vi "SendUDP.vi"(8 "error in (no error)":errorcluster, 11 "data in":string) -> (0 "error out":errorcluster)   [LabVIEW 2013]
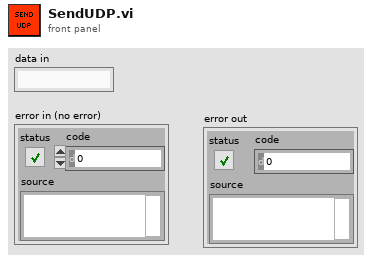
[diagram p1: front panel]
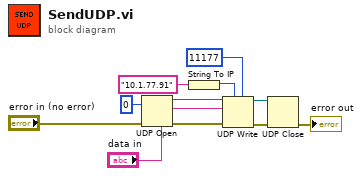
[diagram p0: block diagram]
diagram:
  n1 = UDP Open(8:"error in (no error)", 11:u16 0 ("port")) -> (port=w9:refnum<k16>, 0:w8:errorcluster)  [unwired: 3 in, 1 out]
  n2 = String To IP(1:"10.1.77.91" ("name")) -> (0:w6:u32)
  n3 = UDP Write(address=w6, port or service name=u16 11177 ("port"), connection ID=w9, data in="data in", 8:w8) -> (error out=w3:errorcluster, 3:w2:refnum<k16>)  [unwired: 1 in]
  n4 = UDP Close(connection ID=w2, 8:w3) -> (error out=→"error out":errorcluster)  [unwired: 1 out]
